vi "Read Holding Registers.vi"(6 "timeout ms (1000)":i32=1000, 8 "error in (no error)":errorcluster, 9 "Number of Registers":u16, 10 "Start Address":u16, 11 "TCP Network Connection in":refnum<k5>) -> (0 "error out":errorcluster, 2 "Array":u16[](array[numeric]), 3 "TCP Network Connection out":refnum<k5>)   [LabVIEW 2023, in "Modbus TCP Micro.lvlib"]
uses:
  Modbus TCP Micro.lvlib
  Modbus Functions.ctl
  Modbus Request.vi
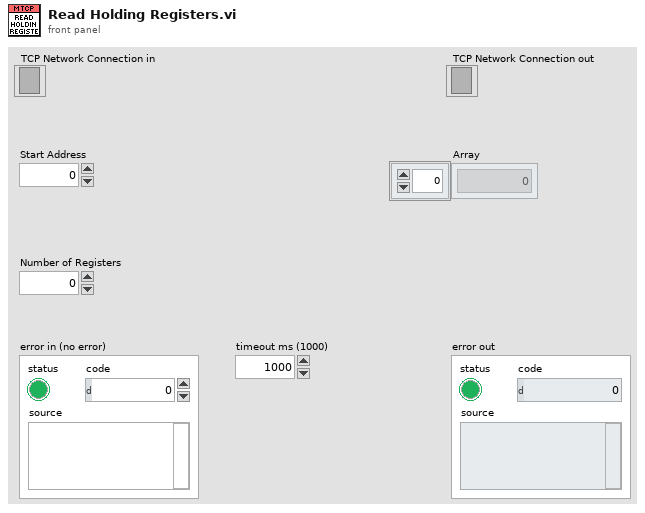
[diagram p1: front panel]
types:
  T1 = typedef "Modbus TCP Micro.lvlib/Modbus Functions.ctl" = u8
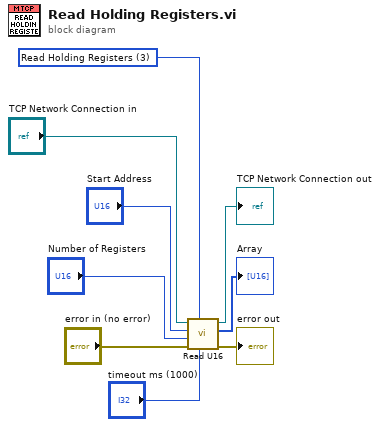
[diagram p0: block diagram]
diagram:
  w2 = T1 3 items=["None"=0, "Read Coil Status"=1, "Read Input Status"=2, "Read Holding Registers"=3, "Read Input Registers"=4, "Force Single Coil"=5, "Preset Single Register"=6, "Force Multiple Coils"=15, "Preset Multiple Registers"=16] ("Function Codes")
  n1 = call "Read U16.vi"("timeout ms (1000)"="timeout ms (1000)", "Function Code"=w2, "error in (no error)"="error in (no error)", "Number of Registers"="Number of Registers", "Start Address"="Start Address", "TCP Network Connection in"="TCP Network Connection in") -> ("error out"=→"error out":errorcluster, "Results"=→"Array":u16[], "TCP Network Connection out"=→"TCP Network Connection out":refnum<k5>)  [unwired: 3 in]
